vi "振动检测.vi"(7 "通道输入":tag="cDAQ2Mod1/ai0", 8 "error in":errorcluster caption="错误输入", 10 "WFGraph引用句柄FFT":refnum<vi>, 11 "WFGraph引用句柄Order":refnum<vi>) -> (0 "error out":errorcluster caption="错误输出", 3 "spectrum info":T1[](array[typedef]) {"x-axis units" items=["Time (s)"=0, "Frequency-CB (Hz)"=1, "Frequency-CPB (Hz)"=1248, "Frequency-Arbitrary (Hz)"=2357, "Quefrency (s)"=2, "Revolutions (rev)"=3, "Order"=4, "Speed (RPM)"=11, "Speed (rad/s)"=21, "Index"=65535]; "weighting filter" items=["Linear", "A-weighting", "B-weighting", "C-weighting", "ITU-R 468-4", "Dolby", "CCITT", "C-message", "Wb", "Wc", "Wd", "We", "Wf", "Wh", "Wj", "Wk", "Wm", "AES17 20 kHz lowpass", "AES17 40 kHz lowpass", "AES17 20 kHz highpass", "AES17 40 kHz highpass"]; "dB reference [EU]" format="%.2f"; "engineering units" items=["custom..."=0, "V"=1, "A"=21, "C"=30, "pC"=31, "s"=32, "-"=29, "Pa"=2, "N"=20, "g"=3, "m/s^2"=4, "m/s"=5, "m"=6, "mm/s"=12, "mm"=13, "micron/s"=14, "micron"=15, "in/s^2"=7, "in/s"=8, "in"=9, "mil/s"=10, "mil"=11, "rad/s^2"=16, "rad/s"=17, "rad"=18, "deg/s^2"=26, "deg/s"=27, "deg"=28, "RPM"=22, "cycle/s^2"=23, "Hz"=24, "cycle"=25, "strain"=19]; "spectral info"."window" items=["None "=0, "Hanning"=1, "Hamming"=2, "Blackman-Harris"=3, "Exact Blackman"=4, "Blackman"=5, "Flat Top"=6, "4 Term B-Harris "=7, "7 Term B-Harris"=8, "Low Sidelobe"=9, "Force - Exponential"=10, "Gaussian"=62]})   [LabVIEW 2020]
uses:
  <vilib>/_NISVFA/_Shared subVIs/Controls/svc_Spectrum Info.ctl
  <vilib>/_NISVFA/_Shared subVIs/Controls/svc_X-Axis Units.ctl
  <vilib>/_NISVFA/_Shared subVIs/Controls/svc_Spectrum Type.ctl
  <vilib>/_NISVFA/_Shared subVIs/Controls/svc_Engineering Units Text Ring.ctl
  <vilib>/_NISVFA/_Shared subVIs/Controls/svc_Weighting Filter Text Ring.ctl
  <vilib>/_NISVFA/_Shared subVIs/Controls/svc_Complimentary Spectrum Units.ctl
panel:
  in  "扫描速率[S/s]":dbl=13500.0 min=0.0 format="%.2f"
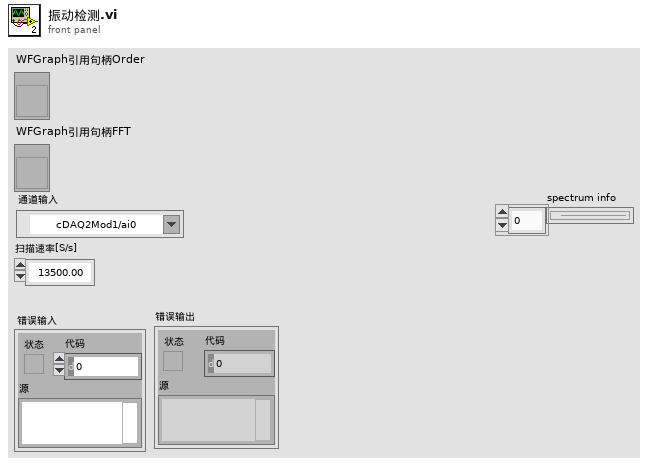
[diagram p1: front panel]
types:
  T1 = typedef "svc_Spectrum Info.ctl" = cluster{"channel name":string, "description":string, "x-axis units":T2, "spectral info":cluster{"spectrum type":T3, "linear/dB":enum16{"linear", "dB"}, "window":u16, "window size":i32, "FFT size":i32}, "engineering units":T4, "custom label":string, "dB reference [EU]":dbl, "peak units":enum16{"rms", "peak", "peak-peak"}, "weighting filter":T5, "spectral density?":bool, "unit label":string, "spectrum skewed?":bool, "complimentary spectrum units":T6}
  T2 = typedef "svc_X-Axis Units.ctl" = u16
  T3 = typedef "svc_Spectrum Type.ctl" = enum16{"FFT Spectrum [complex]", "Amplitude [Magnitude]", "Power [Magnitude^2]", "Cross Spectrum [complex]", "Frequency Response [Complex]"}
  T4 = typedef "svc_Engineering Units Text Ring.ctl" = u16
  T5 = typedef "svc_Weighting Filter Text Ring.ctl" = u16
  T6 = typedef "svc_Complimentary Spectrum Units.ctl" = enum16{"none", "radians", "degrees", "cycles", "imaginary"}
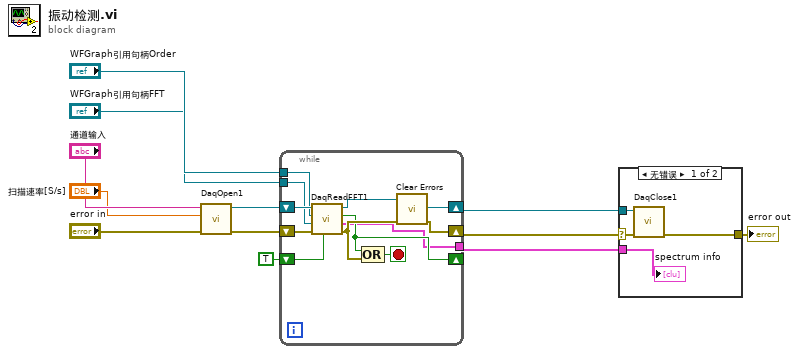
[diagram p0: block diagram]
diagram:
  n1 = call "DaqOpen1.vi"("error in"="error in", "扫描速率[S/s]"="扫描速率[S/s]", "通道输入"="通道输入") -> ("error out"=w5:errorcluster, "task out"=w12:refnum<k21>)  [unwired: 7 in]
  n2 = while {
    tunnel: "WFGraph引用句柄Order" -> [w17]
    tunnel: "WFGraph引用句柄FFT" -> [w19]
    shift-right: [w22] -> w11
    shift-left: w12 -> [w23]
    shift-right: [w15] -> w9
    shift-left: w5 -> [w18]
    shift-right: [w14] -> _
    shift-left: TRUE -> [w16]
    tunnel: [w13] -> w6
    stop <- w20 stop-if-true
    n3 = call "DaqReadFFT1.vi"("restart averaging (F)"=w16, "error in"=w18, "WFGraph引用句柄FFT"=w19, "WFGraph引用句柄Order"=w17, "任务输入"=w23) -> ("error out"=w21:errorcluster, "spectrum info"=w13:T1[], "done"=w14:bool, "task out 2"=w22:refnum<k21>)  [unwired: 3 in]
    n4 = Compound Arithmetic op=OR ("复合运算")(w14, w21) -> (w20:bool)
    n5 = call <vilib>:"Clear Errors.vi"("error in (no error)"=w21) -> ("error out"=w15:errorcluster)  [unwired: 5 in, 1 out]
  }
  n6 = case shown="无错误" w9 {
    selector: w9 -> [w26 w28]
    tunnel: w11 -> [w27 _]
    tunnel: [w25 w28] -> w8
    tunnel: w6 -> [w24 _]
    frame No Error {
      n7 = call "DaqClose1.vi"("error in"=w26, "task in"=w27) -> ("error out"=w25:errorcluster)  [unwired: 9 in]
      "spectrum info" <- w24
    }
    frame Error {
    }
  }
  "error out" <- w8
